vi "return.vi"(2 "y in":i32) -> (0 "y out":i32, 1 "Enum":T1(ring))   [LabVIEW 2016]
uses:
  <vilib>/NXT/Block Support/NXT_OutputPort.ctl
  <vilib>/NXT/NXTIO Xnodes/NXTIONodeSubVIs/NXTStopMotors.vi
  <vilib>/NXT/NXTIO Xnodes/NXTIONodeSubVIs/NXTMotorRunDistance.vi
  <vilib>/NXT/NXTIO Xnodes/NXTIONodeSubVIs/LEGOMotorStatus.vi
  <vilib>/NXT/NXTIO Xnodes/NXTIONodeSubVIs/NXTMoveMotors.vi
  <vilib>/NXT/NXTIO Xnodes/NXTIONodeSubVIs/LEGOResetMotors.vi
  <vilib>/NXT/Subs/LVHSConnector.ctl
  <vilib>/NXT/NXTIO Xnodes/AddressXNode/NXTIOAddress.xnode
  <vilib>/NXT/NXTIO Xnodes/NXTIOXNode/NXTIO.xnode
  <vilib>/NXT/LegoClasses/BrickReference/BrickReference.lvclass
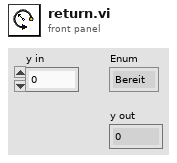
[diagram p1: front panel]
types:
  T1 = enum16{"Bereit", "Move 1", "Reference_pos", "Wait", "row1_check", "row2_check", "row3_check", "return", "move2", "move3", "move4", "move5", "end"}
  T2 = typedef "NXT_OutputPort.ctl" = u8
  T3 = cluster{"Output Port":T2, "Output Port 2":T2, "Output Port 3":T2}
  T4 = typedef "LVHSConnector.ctl" = refnum<class "BrickReference.lvclass">
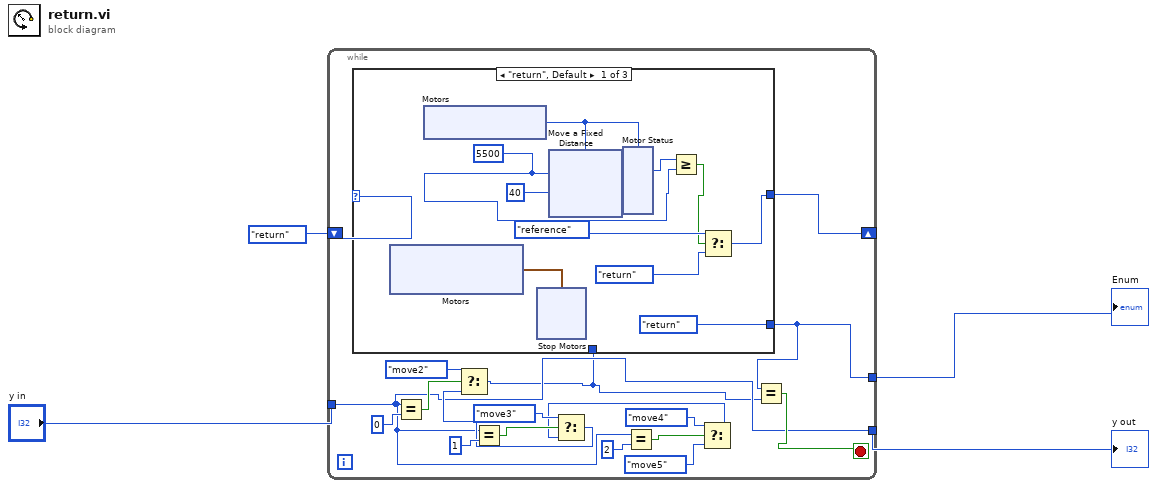
[diagram p0: block diagram]
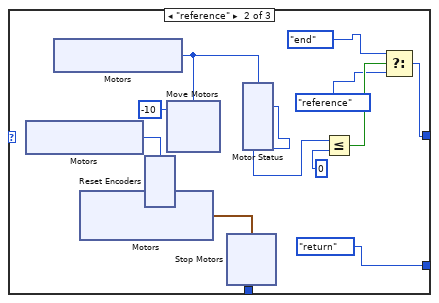
[diagram p2: hidden frame]
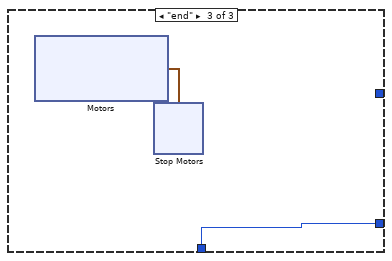
[diagram p3: hidden frame]
diagram:
  n1 = while {
    shift-right: [w21] -> _
    shift-left: enum16{"return", "reference", "end"}."return" -> [w22]
    tunnel: [w8] -> w1
    tunnel: "y in" -> [w6]
    tunnel: [w6] -> w4
    stop <- w7 stop-if-true
    n2 = Equal?(x=w6, y=0) -> (x = y?=w19:bool)
    n3 = Equal?(x=w6, y=1) -> (x = y?=w16:bool)
    n4 = Equal?(x=w6, y=2) -> (x = y?=w13:bool)
    n5 = Select(t=T1."move4", s=w13, f=T1."move5") -> (s? t:f=w11:T1)
    n6 = Select(t=T1."move3", s=w16, f=w11) -> (s? t:f=w10:T1)
    n7 = Select(t=T1."move2", s=w19, f=w10) -> (s? t:f=w5:T1)
    n8 = case shown="\"return\", Default" w22 {
      tunnel: [w26 w61 _] -> w21
      tunnel: [T1."return" T1."return" w97] -> w8
      tunnel: w5 -> [_ _ w97]
      frame "return", Default {
        w24 = 5500 ("Distance 1")
        n9 = xnode "Motors"() -> ("Motor"=w33:cluster{"Port":T2, "Port":T2})
        n10 = xnode "Motors"() -> ("Motor"=w30:T2)
        n11 = xnode "Stop Motors"("Motors"=w33) -> ()  [unwired: 1 in, 1 out]
        n12 = xnode "Move a Fixed Distance"("Speed 1"=i8 40, "Distance 1"=w24, "Motors"=w30) -> ("NXT/EV3"=w29:T4)  [unwired: 1 in]
        n13 = xnode "Motor Status"("Motors"=w30, "NXT/EV3"=w29) -> ("Position 1"=w25:i32)  [unwired: 2 out]
        n14 = Greater Or Equal?(x=w25, y=w24) -> (x >= y?=w23:bool)
        n15 = Select(t=enum16{"return", "reference", "end"}."reference", s=w23, f=enum16{"return", "reference", "end"}."return") -> (s? t:f=w26:enum16{"return", "reference", "end"})
      }
      frame "reference" {
        n16 = xnode "Motors"() -> ("Motor"=w59:T2)
        n17 = xnode "Motors"() -> ("Motor"=w65:T2)
        n18 = xnode "Motors"() -> ("Motor"=w68:cluster{"Port":T2, "Port":T2})
        n19 = xnode "Reset Encoders"("Motors"=w59) -> ()  [unwired: 1 in, 1 out]
        n20 = xnode "Move Motors"("Power/Speed 1"=i8 -10, "Motors"=w65) -> ()  [unwired: 1 in, 1 out]
        n21 = xnode "Stop Motors"("Motors"=w68) -> ()  [unwired: 1 in, 1 out]
        n22 = xnode "Motor Status"("Motors"=w65) -> ("Position 1"=w67:i32)  [unwired: 1 in, 2 out]
        n23 = Less Or Equal?(x=w67, y=0) -> (x <= y?=w66:bool)
        n24 = Select(t=enum16{"return", "reference", "end"}."end", s=w66, f=enum16{"return", "reference", "end"}."reference") -> (s? t:f=w61:enum16{"return", "reference", "end"})
      }
      frame "end" {
        n25 = xnode "Motors"() -> ("Motor"=w98:cluster{"Port":T2, "Port":T2, "Port":T2})
        n26 = xnode "Stop Motors"("Motors"=w98) -> ()  [unwired: 1 in, 1 out]
      }
    }
    n27 = Equal?(x=w8, y=w5) -> (x = y?=w7:bool)
  }
  "y out" <- w4
  "Enum" <- w1
